vi "Launch Two Common Measurements.vi"() -> ()   [LabVIEW 2015]
uses:
  Libraries/Mag Lab Measure/Common Measurements/Load App.vi
  Libraries/Mag Lab Measure/Common Measurements/Common Measurements.lvclass
panel:
  out "Current action two:":string
  out "Waiting Lights":T1
  out "Current action one:":string
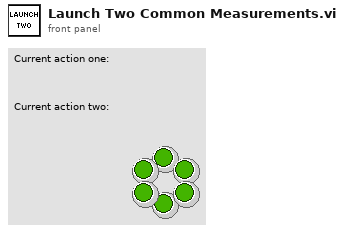
[diagram p1: front panel]
types:
  T1 = cluster{"DNL_wait 1":bool, "DNL_wait 1":bool, "DNL_wait 1":bool, "DNL_wait 1":bool, "DNL_wait 1":bool, "DNL_wait 1":bool}
  T2 = cluster{"[0]":bool, "[1]":bool, "[2]":bool, "[3]":bool, "[4]":bool, "[5]":bool}
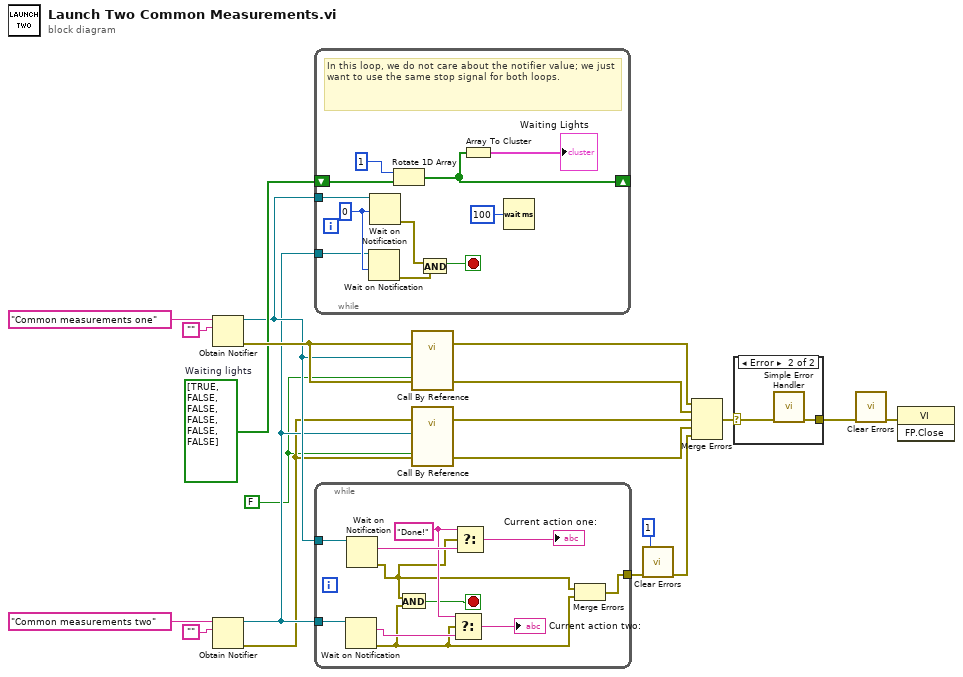
[diagram p0: block diagram]
diagram:
  w12 = bool[] [TRUE, FALSE, FALSE, FALSE, FALSE, FALSE]  # Waiting lights
  w6 = FALSE ("Open Actor Core front panel? (F)")
  n1 = Obtain Notifier(name (unnamed)="Common measurements one", notification data type="") -> (notifier out=w11:refnum<notifier>, error out=w16:errorcluster)  [unwired: 2 in, 1 out]
  n2 = Obtain Notifier(name (unnamed)="Common measurements two", notification data type="") -> (notifier out=w8:refnum<notifier>, error out=w7:errorcluster)  [unwired: 2 in, 1 out]
  n3 = while {
    shift-right: [w26] -> _
    shift-left: w12 -> [w28]
    tunnel: w11 -> [w30]
    tunnel: w8 -> [w21]
    stop <- w24 stop-if-true
    w22 = 0 ("timeout in ms (-1)")
    # "In this loop, we do not care about the notifier value; we just want to use the same stop signal for both loops."
    n4 = Wait on Notification(notifier=w21, timeout in ms (-1)=w22) -> (error out=w23:errorcluster)  [unwired: 2 in, 3 out]
    n5 = Wait on Notification(notifier=w30, timeout in ms (-1)=w22) -> (error out=w31:errorcluster)  [unwired: 2 in, 3 out]
    n6 = Rotate 1D Array(1:w28, 2:1 ("n")) -> (0:w26:bool[])
    n7 = And(x=w31, y=w23) -> (x .and. y?=w24:bool)
    n8 = Array To Cluster(array=w26) -> (cluster=→"Waiting Lights":T2)
    n9 = Wait (ms)(milliseconds to wait=u32 100) -> ()  [unwired: 1 out]
  }
  n10 = while {
    tunnel: w11 -> [w42]
    tunnel: [w36] -> w3
    tunnel: w8 -> [w39]
    stop <- w34 stop-if-true
    w38 = "Done!" ("notification")
    n11 = Wait on Notification(notifier=w39) -> (notification=w37:string, error out=w32:errorcluster)  [unwired: 3 in, 2 out]
    n12 = Wait on Notification(notifier=w42) -> (notification=w41:string, error out=w35:errorcluster)  [unwired: 3 in, 2 out]
    n13 = And(x=w35, y=w32) -> (x .and. y?=w34:bool)
    n14 = Select(t=w38, s=w32, f=w37) -> (s? t:f=→"Current action two:":string)
    n15 = Select(t=w38, s=w35, f=w41) -> (s? t:f=→"Current action one:":string)
    n16 = Merge Errors(w35, w32) -> (w36:errorcluster)
  }
  n17 = call-by-ref "?"(error in=w16, "Open Actor Core front panel? (F)"=w6, "Error In"=w16, "Status Notifier"=w11) -> (error out=w18:errorcluster, "Error Out"=w15:errorcluster)  [unwired: 9 in, 1 out]
  n18 = call-by-ref "?"(error in=w7, "Open Actor Core front panel? (F)"=w6, "Error In"=w7, "Status Notifier"=w8) -> (error out=w5:errorcluster, "Error Out"=w4:errorcluster)  [unwired: 9 in, 1 out]
  n19 = call <vilib>:"Clear Errors.vi"("error in (no error)"=w3, "specific error code to clear (0: all)"=1) -> ("error out"=w2:errorcluster)  [unwired: 4 in, 1 out]
  n20 = Merge Errors(w18, w15, w5, w4, w2) -> (w19:errorcluster)
  n21 = case shown="Error" w19 {
    selector: w19 -> [w43 w45]
    tunnel: [w43 w44] -> w13
    frame No Error {
    }
    frame Error {
      n22 = call <vilib>:"Simple Error Handler.vi"("error in (no error)"=w45) -> ("error out"=w44:errorcluster)  [unwired: 4 in, 4 out]
    }
  }
  n23 = call <vilib>:"Clear Errors.vi"("error in (no error)"=w13) -> ("error out"=w20:errorcluster)  [unwired: 5 in, 1 out]
  n24 = invoke class="VI" method="FP.Close"(error in=w20) -> ()  [unwired: 2 in, 3 out]
